vi "Close Front Panel.vi"(8 "error in (no error)":errorcluster, 10 "View Hierarchy Level":i32, 11 "GUI View Actor in":refnum<class "GUI View Actor.lvclass">) -> (0 "error out":errorcluster, 3 "GUI View Actor out":refnum<class "GUI View Actor.lvclass">)   [LabVIEW 2017, in "GUI Views.lvlib" / "GUI View Actor.lvclass"]
doc: "Closes the Front Panel of a specified Actor Core VI of the the specified View class hierarchy. The method is active only if the GUI View is not contained. The Front Panel is specified by: \n\n<b> View Hierarchy Level</b> the level on the subclassing hierarchy of the GUI View actor, it is used to choose the Actor Core Front Panel among all the exisiting sublcasses of the GUI VIew Actor present in the View specified above"
uses:
  GUI View Actor.lvclass
  GUI View Actor.lvclass/GUI View Actor.ctl
  properties/Read Managed by Container.vi
  <vilib>/ActorFramework/Message Enqueuer/Equals Not A Refnum.vi
  <vilib>/ActorFramework/Message Enqueuer/Message Enqueuer.lvclass
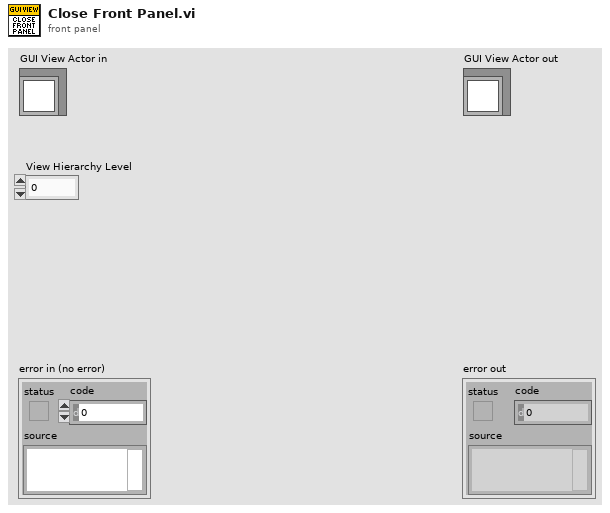
[diagram p1: front panel]
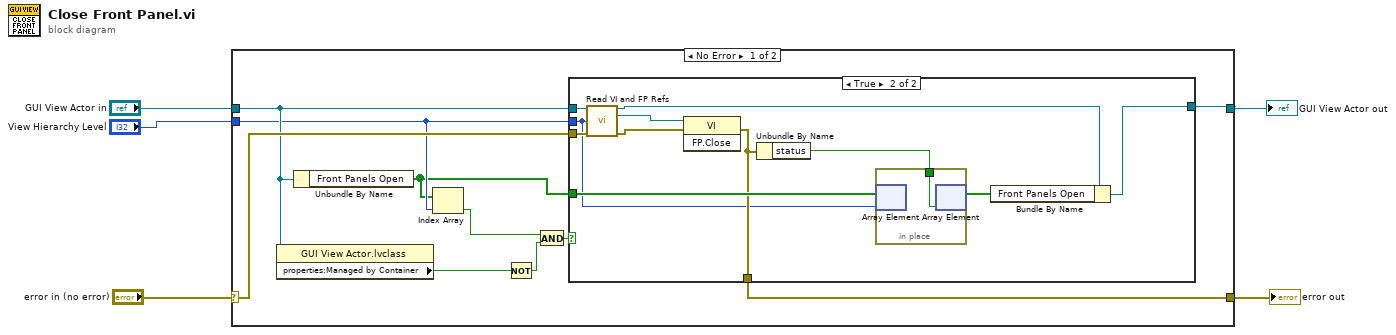
[diagram p0: block diagram]
diagram:
  n1 = case shown="No Error" "error in (no error)" {
    selector: "error in (no error)" -> [w15 w31]
    tunnel: [w13 w31] -> w4
    tunnel: [w14 w30] -> w2
    tunnel: "GUI View Actor in" -> [w11 w30]
    tunnel: "View Hierarchy Level" -> [w7 _]
    frame No Error {
      n2 = property class="GUI View Actor.lvclass"(reference=w11) -> ("properties:Managed by Container"=w12:bool)  [unwired: 1 in, 2 out]
      n3 = Unbundle By Name(w11) -> ("Front Panels Open"=w6:bool[])
      n4 = Index Array(array=w6, index=w7) -> (element=w9:bool)
      n5 = Not(x=w12) -> (.not. x?=w10:bool)
      n6 = And(x=w9, y=w10) -> (x .and. y?=w8:bool)
      n7 = case shown="True" w8 {
        tunnel: w15 -> [w16 w27]
        tunnel: w7 -> [_ w18]
        tunnel: [w17 w20] -> w14
        tunnel: [w16 w22] -> w13
        tunnel: w11 -> [w17 w24]
        tunnel: w6 -> [_ w23]
        frame False {
        }
        frame True {
          n8 = call "Read VI and FP Refs.vi"("GUI View Actor in"=w24, "View Hierarchy Level"=w18, "error in (no error)"=w27) -> ("GUI View Actor out"=w25:refnum<class "GUI View Actor.lvclass">, "VI Ref"=w28:refnum<vi>, "error out"=w26:errorcluster)  [unwired: 8 in, 2 out]
          n9 = invoke class="VI" method="FP.Close"(reference=w28, error in=w26) -> (error out=w22:errorcluster)  [unwired: 1 in, 2 out]
          n10 = Unbundle By Name(w22) -> ("status"=w21:bool)
          n11 = in-place {
            in-place-border: w21 -> [w29]
            n12 = in-place-array #1(w23, w18) -> ()  [unwired: 1 out]
            n13 = in-place-array #1(w29) -> (w19:bool[])  [unwired: 1 out]
          }
          n14 = Bundle By Name(cluster=w25, "Front Panels Open"=w19) -> (w20:refnum<class "GUI View Actor.lvclass">)
        }
      }
    }
    frame Error {
    }
  }
  "error out" <- w4
  "GUI View Actor out" <- w2
